vi "Write Data Model.vi"(8 "error in":errorcluster, 10 "Device Data Model":refnum<class "Device Data Model.lvclass">, 11 "Modbus slave in":refnum<class "Modbus Slave.lvclass">) -> (0 "error out":errorcluster, 3 "Modbus slave out":refnum<class "Modbus Slave.lvclass">)   [LabVIEW 2015, in "Modbus Library.lvlib" / "Modbus Slave.lvclass"]
doc: "This VI is an accessor for the <B>data model</B> stored in the Modbus master instance. This accessor can be used as a property node. This model defines how the slave stores data and reacts to functions and data sent by a Modbus master. This function closes the original data model stored."
uses:
  Modbus Slave.lvclass
  Data Model/Device Data Model.lvclass
  Modbus Slave.lvclass/Modbus Slave.ctl
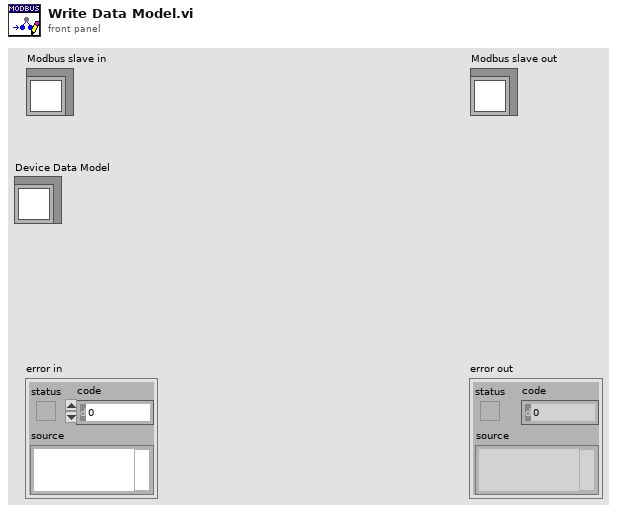
[diagram p1: front panel]
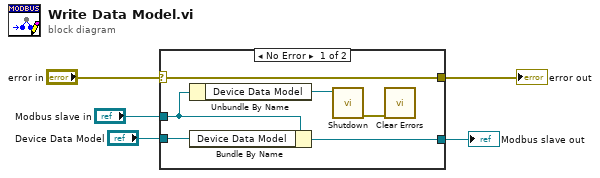
[diagram p0: block diagram]
diagram:
  n1 = case shown="No Error" "error in" {
    selector: "error in" -> [w11 w12]
    tunnel: [w11 w12] -> w4
    tunnel: [w10 w13] -> w2
    tunnel: "Modbus slave in" -> [w9 w13]
    tunnel: "Device Data Model" -> [w8 _]
    frame No Error {
      n2 = Unbundle By Name(w9) -> ("Device Data Model"=w7:refnum<class "Device Data Model.lvclass">)
      n3 = Bundle By Name(cluster=w9, "Device Data Model"=w8) -> (w10:refnum<class "Modbus Slave.lvclass">)
      n4 = call-dynamic "Shutdown.vi"("device data model in"=w7) -> ("error out"=w6:errorcluster)  [unwired: 10 in]
      n5 = call <vilib>:"Clear Errors.vi"("error in (no error)"=w6) -> ()  [unwired: 5 in, 2 out]
    }
    frame Error {
    }
  }
  "error out" <- w4
  "Modbus slave out" <- w2
